vi "Node.vi"(8 "error in (no error)":errorcluster, 11 "Node Ptr":T1 format="%.0x") -> (0 "error out":errorcluster)   [LabVIEW 2016, in "PXImc Custom Device System Explorer.lvlib"]
uses:
  PXImc Custom Device System Explorer.lvlib
  <vilib>/NI Veristand/Custom Device API/Custom Device Item Ref.ctl
  Shared/Constants.vi
  <vilib>/NI Veristand/Custom Device API/Get Item Property (Variant).vi
  <vilib>/NI Veristand/Custom Device API/Set Item Property (Variant).vi
  <vilib>/NI VeriStand/Custom Device API/Custom Device API.lvlib
  Shared/PXImc Custom Device Shared.lvlib
panel:
  out "Imported Channels":string[][](table)
  out "Local Channels":string[][](table)
  out "PXImc Resource Name":string
  in  "Connection Timeout (s)":dbl
  in  "Readers Buffer Size":u64
  in  "Configution Files Path":path
  in  "Update Configuration":bool
  in  "Header":cluster{"Section Name":string}={"Section Name"="Custom Device Item Settings"}
  in  "Description":string
  in  "Name":string
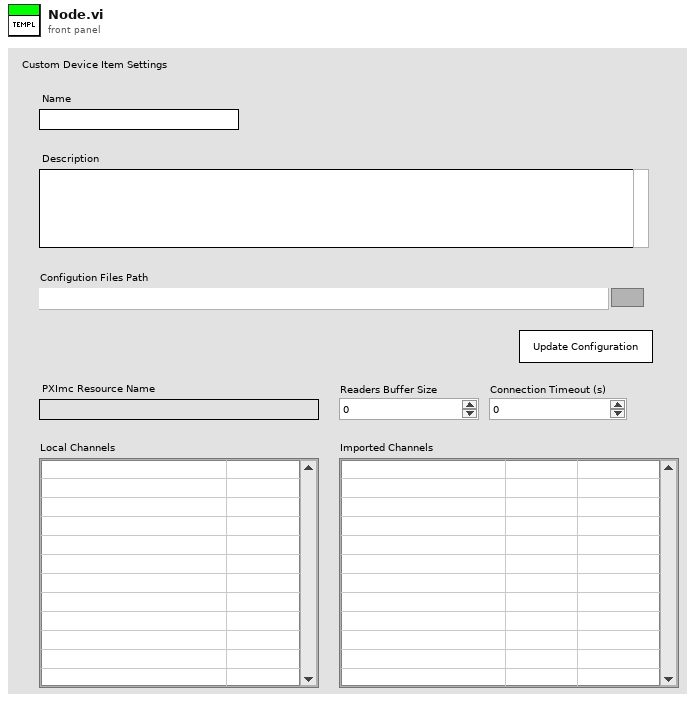
[diagram p1: front panel]
types:
  T1 = typedef "Custom Device API.lvlib/Custom Device Item Ref.ctl" = u64
  T2 = typedef "Custom Device API.lvlib/Custom Device Item Info.ctl" = cluster{"Name":string, "Is Channel":bool, "GUID":string, "Is Waveform":bool}
  T3 = typedef "PXImc Custom Device Shared.lvlib/Compiled.Settings.ctl" = cluster{"Target Type":T4, "Router Properties":T5, "Node Data":T10, "Configuration Folder Path":path}
  T4 = typedef "PXImc Router.lvlib/Target Type.ctl" = enum16{"Router", "Node"}
  T5 = typedef "PXImc Router.lvlib/Router - Configuration.ctl" = cluster{"Target Type":T4, "Master Table Ref":refnum<data-value>, "Master Table Size (Bytes)":u32, "Node Properties":T6[], "Router - PXImc Properties":T8}
  T6 = typedef "PXImc Router.lvlib/Node Block R-W Properties.ctl" = cluster{"Node ID":u32, "# Reading Blocks":u32, "Node Writing Block":T7, "Node Reading Blocks":T7[]}
  T7 = typedef "PXImc Router.lvlib/Block Properties.ctl" = cluster{"Offset":u32, "Size (Bytes)":u32}
  T8 = typedef "PXImc Router.lvlib/Router - PXImc Properties.ctl" = cluster{"PXImc Cards Properties":T9[], "Connection Timeout (s)":dbl, "Readers Buffer Size":u64}
  T9 = typedef "PXImc Router.lvlib/Router - PXImc Card Properties.ctl" = cluster{"PXImc Resource Name":string, "Reader - PXImc Session Ref":refnum<k21>, "Writer - PXImc Session Ref":refnum<k21>, "Reader Conn ID":u16, "Writer Conn ID":u16}
  T10 = typedef "PXImc Router.lvlib/Node Data.ctl" = cluster{"Node Name":string, "PXImc Parameters":T11, "Local Data":T12, "Imported Data":T15}
  T11 = typedef "PXImc Router.lvlib/Node - PXImc Parameters.ctl" = cluster{"Resource Name":string, "Connection Timeout (s)":dbl, "Readers Buffer Size":u64, "Node PXImc Reader Conn Id":u16, "Node PXImc Writer Conn Id":u16, "Writer PXImc Session":refnum<k21>, "Reader PXImc Session":refnum<k21>}
  T12 = typedef "PXImc Router.lvlib/Node - Writer Data.ctl" = cluster{"Noder ID":u32, "Byte Buffer Ref":refnum<class "Byte Buffer.lvclass">, "Master Table Offest":u32, "Byte Buffer Size":u32, "Node Local Channels":T13[], "Node Local Channels Table":string[][]}
  T13 = typedef "PXImc Router.lvlib/Node Ch Properties.ctl" = cluster{"Name":string, "Value":dbl, "Data Type":T14}
  T14 = typedef "PXImc Router.lvlib/Data Type.ctl" = enum16{"Boolean", "SGL", "DBL", "I8", "I16", "I32", "I64", "U8", "U16", "U32", "U64"}
  T15 = typedef "PXImc Router.lvlib/Node - Readers Data.ctl" = cluster{"Byte Buffer Ref":refnum<class "Byte Buffer.lvclass">, "Byte Buffer Size":u64, "Readers Data Array":T16[], "Node Imported Channels Table":string[][]}
  T16 = typedef "PXImc Router.lvlib/Node - Reader Data.ctl" = cluster{"Noder ID":u32, "Master Table Offest":u32, "Byte Buffer Size":u64, "Node Imported Channels":T13[]}
  T17 = typedef "Custom Device API.lvlib/Custom Device Commands.ctl" = enum16{"Default", "Item renamed", "Shutdown", "Dynamic button pressed"}
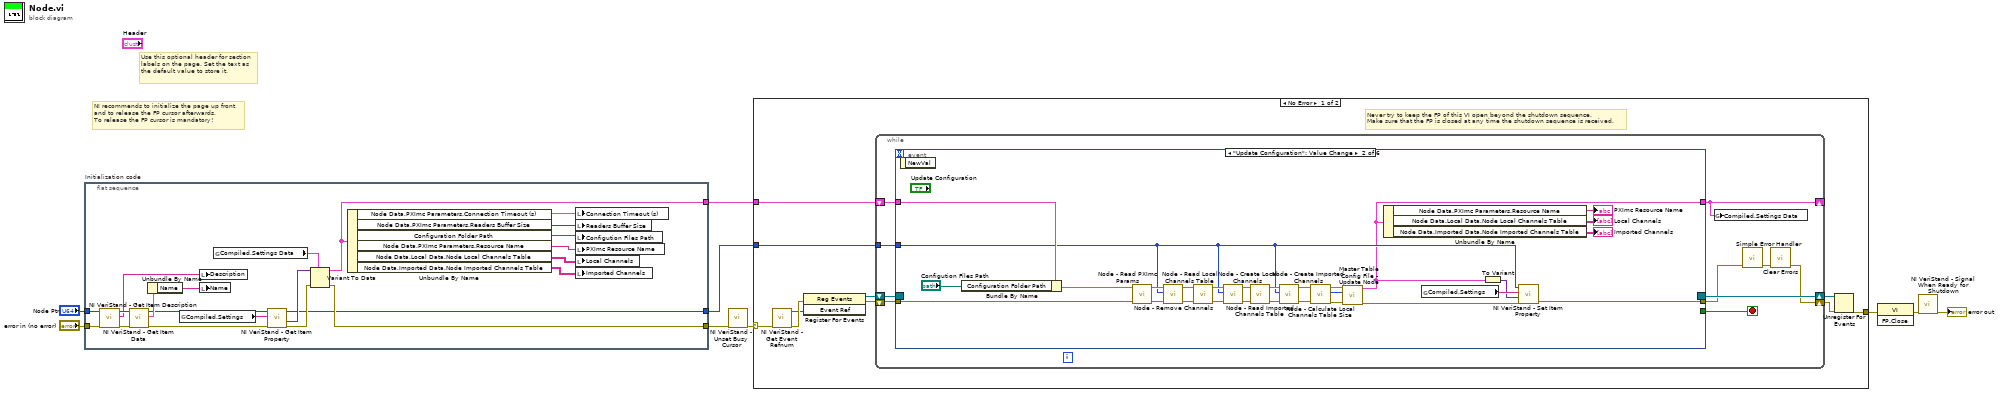
[diagram p0: block diagram]
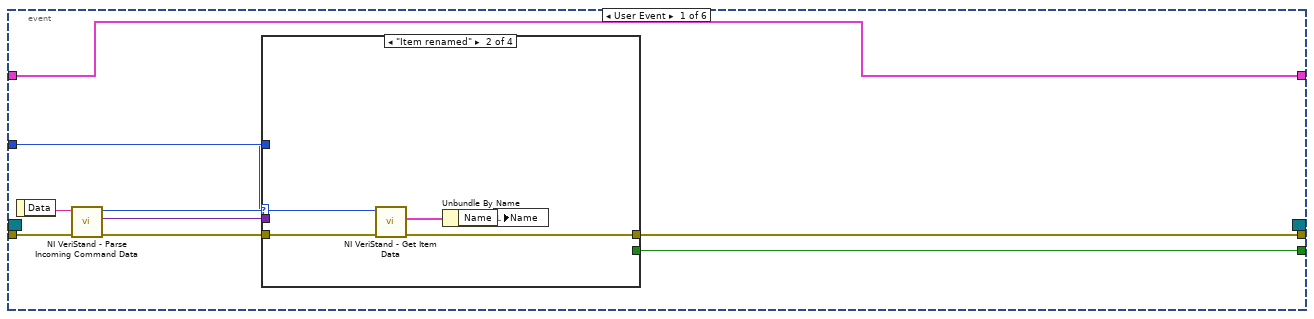
[diagram p2: hidden frame]
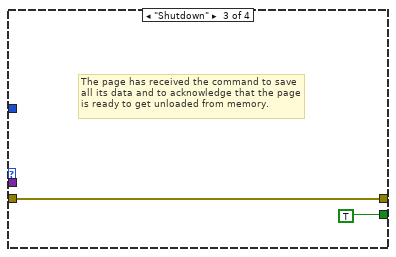
[diagram p4: hidden frame]
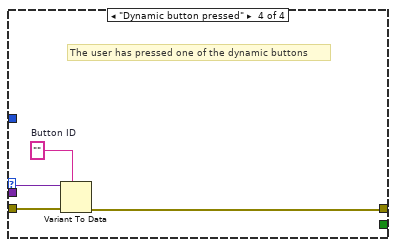
[diagram p5: hidden frame]
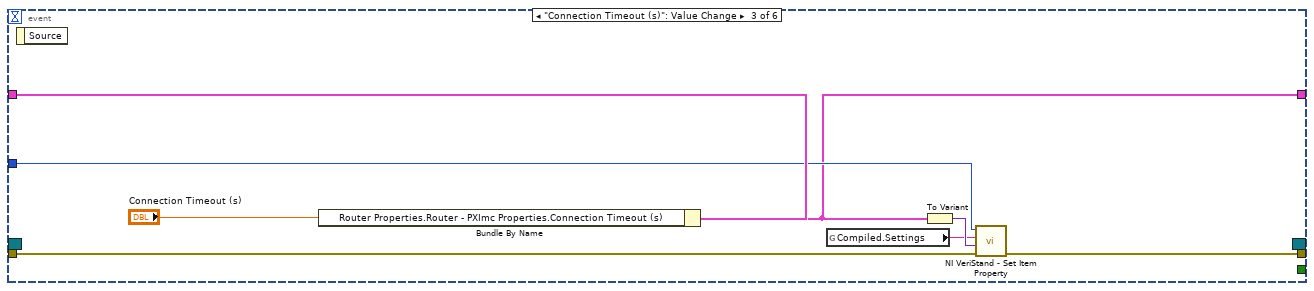
[diagram p6: hidden frame]
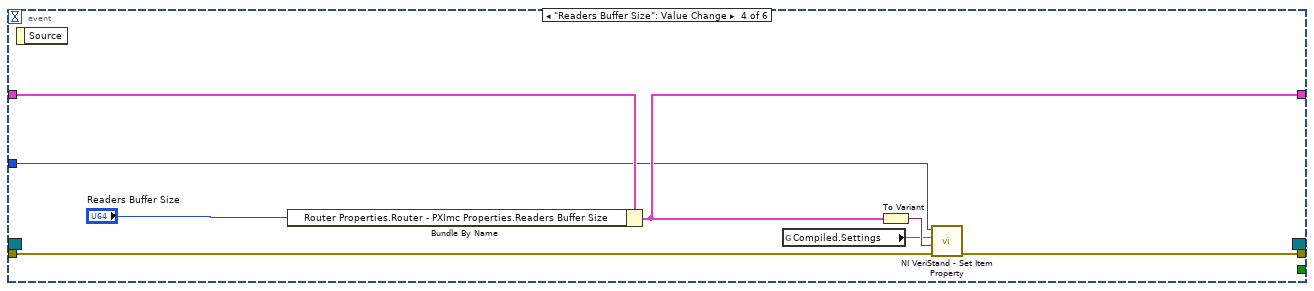
[diagram p7: hidden frame]
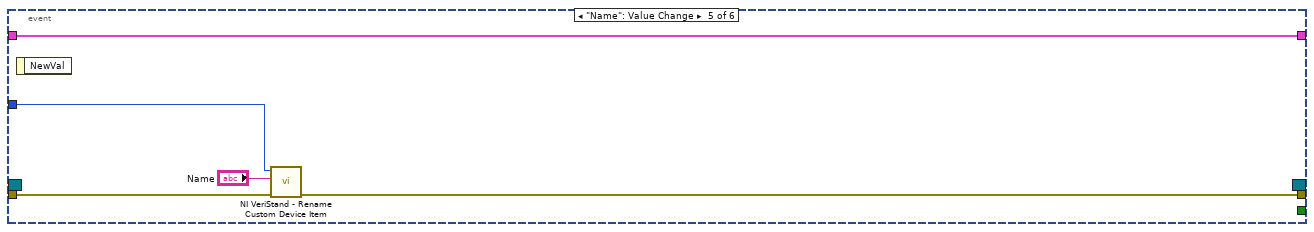
[diagram p8: hidden frame]
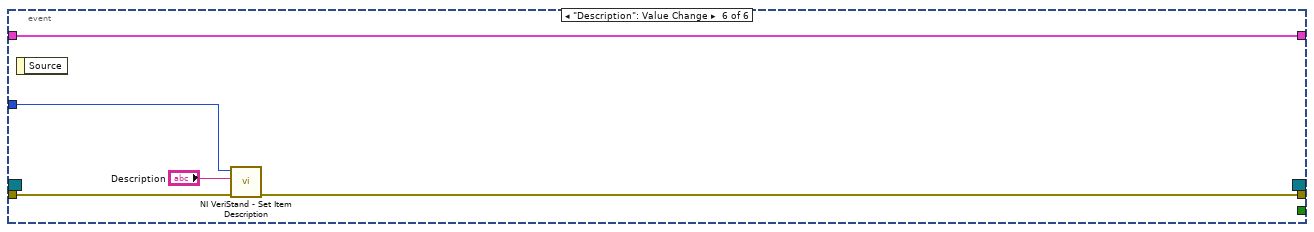
[diagram p9: hidden frame]
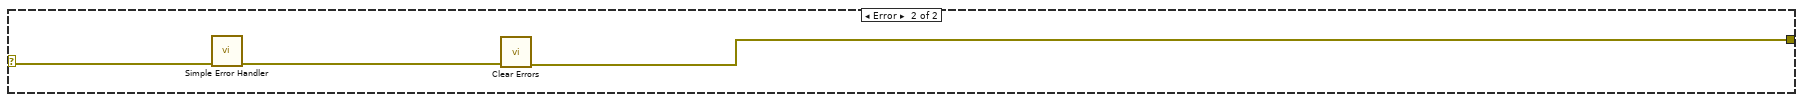
[diagram p10: hidden frame]
diagram:
  # "Use this optional header for section labels on the page. Set the text as the default value to store it."
  # "NI recommends to initialize the page up front\nand to release the FP cursor afterwards.\nTo release the FP cursor is mandatory!"
  n1 = flat-sequence "Initialization code" {
    tunnel: "error in (no error)" -> [w30]
    tunnel: "Node Ptr" -> [w29]
    tunnel: [w16] -> w5
    tunnel: [w15] -> w2
    tunnel: [w14] -> w1
    frame #0 {
      n2 = call <vilib>:"NI VeriStand - Get Item Description.vi"("error in (no error)"=w30, "Item Ref in"=w29) -> ("error out"=w27:errorcluster, "Description"=w28:string, "Item Ref out"=w31:T1)  [unwired: 7 out]
      n3 = call <vilib>:"NI VeriStand - Get Item Data.vi"("error in (no error)"=w27, "Item Ref in"=w31) -> ("error out"=w17:errorcluster, "Item Info"=w26:T2, "Item Ref out"=w18:T1)  [unwired: 7 out]
      n4 = Unbundle By Name(w26) -> ("Name"=w13:string)
      n5 = global read "Constants.vi" "Compiled.Settings"() -> (w19:string)
      n6 = local write "Description"(w28) -> ()
      n7 = local write "Name"(w13) -> ()
      n8 = global read "Constants.vi" "Compiled.Settings Data"() -> (w12:T3)
      n9 = call-poly <vilib>:"NI VeriStand - Get Item Property.vi"("error in (no error)"=w17, "Property Name"=w19, "Item Ref in"=w18) -> ("error out"=w20:errorcluster, "Value"=w21:variant, "Item Ref out"=w15:T1)  [unwired: 5 in, 1 out]
      n10 = Variant To Data(error in=w20, type=w12, Variant=w21) -> (data=w14:T3, error out=w16:errorcluster)
      n11 = Unbundle By Name(w14) -> ("Node Data.PXImc Parameters.Connection Timeout (s)"=w22:dbl, "Node Data.PXImc Parameters.Readers Buffer Size"=w23:u64, "Configuration Folder Path"=w24:path, "Node Data.PXImc Parameters.Resource Name"=w25:string, "Node Data.Local Data.Node Local Channels Table"=w11:string[][], "Node Data.Imported Data.Node Imported Channels Table"=w10:string[][])
      n12 = local write "Connection Timeout (s)"(w22) -> ()
      n13 = local write "Readers Buffer Size"(w23) -> ()
      n14 = local write "Configution Files Path"(w24) -> ()
      n15 = local write "PXImc Resource Name"(w25) -> ()
      n16 = local write "Local Channels"(w11) -> ()
      n17 = local write "Imported Channels"(w10) -> ()
    }
  }
  n18 = call <vilib>:"NI VeriStand - Unset Busy Cursor.vi"("error in (no error)"=w5) -> ("error out"=w4:errorcluster)  [unwired: 10 out]
  n19 = case shown="No Error" w4 {
    selector: w4 -> [w33 w129]
    tunnel: [w38 w127] -> w9
    tunnel: w2 -> [w34 _]
    tunnel: w1 -> [w32 _]
    frame No Error {
      # "Never try to keep the FP of this VI open beyond the shutdown sequence.\nMake sure that the FP is closed at any time the shutdown sequence is received."
      n20 = call <vilib>:"NI VeriStand - Get Event Refnum.vi"("error in (no error)"=w33) -> ("error out"=w41:errorcluster, "Event Ref"=w37:refnum<user-event>)  [unwired: 9 out]
      n21 = register-events(error in=w41, w37) -> (reference out=w35:refnum<event-registration>, error out=w36:errorcluster)  [unwired: 1 in]
      n22 = while {
        tunnel: w34 -> [w47]
        shift-right: [w44] -> w39
        shift-left: w36 -> [w50]
        shift-right: [w51] -> w40
        shift-left: w35 -> [w49]
        shift-right: [w42] -> _
        shift-left: w32 -> [w43]
        stop <- w48 stop-if-true
        n23 = event shown="[1] \"Update Configuration\": Value Change" {
          selector: w49 -> [_ _ _ _ _ _]
          dyn-events: [_ _ _ _ _ _] -> w51
          timeout: _ -> [_ _ _ _ _ _]
          tunnel: w50 -> [w60 w93 w103 w110 w121 w125]
          tunnel: [w56 _ _ _ _ _] -> w48
          tunnel: [w55 w98 w102 w109 w120 w124] -> w46
          tunnel: w47 -> [w54 w82 w104 w111 w119 w126]
          tunnel: w43 -> [w52 w97 w106 w114 w117 w122]
          tunnel: [w52 w74 w101 w112 w117 w122] -> w42
          event User Event {
            n24 = event-data() -> ("Data"=w59:string)  [unwired: 1 out]
            n25 = call <vilib>:"NI VeriStand - Parse Incoming Command Data.vi"("error in (no error)"=w60, "Incoming data"=w59) -> ("error out"=w58:errorcluster, "Outgoing data"=w53:variant, "Action"=w57:T17)  [unwired: 7 out]
            n26 = case shown="\"Item renamed\"" w57 {
              tunnel: w58 -> [w61 w66 w67 w72]
              tunnel: [_ _ TRUE _] -> w56
              tunnel: [w61 w63 w67 w69] -> w55
              tunnel: w54 -> [_ w65 _ _]
              tunnel: w53 -> [_ _ _ w71]
              frame "Default", Default {
              }
              frame "Item renamed" {
                n27 = call <vilib>:"NI VeriStand - Get Item Data.vi"("error in (no error)"=w66, "Item Ref in"=w65) -> ("error out"=w63:errorcluster, "Item Info"=w64:T2)  [unwired: 8 out]
                n28 = Unbundle By Name(w64) -> ("Name"=w62:string)
                n29 = local write "Name"(w62) -> ()
              }
              frame "Shutdown" {
                # "The page has received the command to save all its data and to acknowledge that the page is ready to get unloaded from memory."
              }
              frame "Dynamic button pressed" {
                w70 = ""  # Button ID
                # "The user has pressed one of the dynamic buttons"
                n30 = Variant To Data(error in=w72, type=w70, Variant=w71) -> (error out=w69:errorcluster)  [unwired: 1 out]
              }
            }
          }
          event "Update Configuration": Value Change {
            n31 = event-data() -> ()  [unwired: 2 out]
            n32 = Bundle By Name(cluster=w97, "Configuration Folder Path"="Configution Files Path") -> (w94:T3)
            n33 = call "Node - Read PXImc Params.vi"("error in (no error)"=w93, "Compiled.Settings In"=w94) -> ("error out"=w81:errorcluster, "Compiled.Settings Out"=w84:T3)  [unwired: 8 in]
            n34 = call "Node - Remove Channels.vi"("error in (no error)"=w81, "Node Ptr In"=w82, "Compiled.Settings In"=w84) -> ("error out"=w80:errorcluster, "Compiled.Settings Out"=w83:T3)  [unwired: 6 in, 1 out]
            n35 = call "Node - Read Local Channels Table.vi"("error in (no error)"=w80, "Compiled.Settings In"=w83) -> ("error out"=w91:errorcluster, "Compiled.Settings Out"=w92:T3)  [unwired: 8 in]
            n36 = call "Node - Create Local Channels.vi"("error in (no error)"=w91, "Node Ptr In"=w82, "Compiled.Settings In"=w92) -> ("error out"=w89:errorcluster, "Compiled.Settings Out"=w90:T3)  [unwired: 6 in, 1 out]
            n37 = call "Node - Read Imported Channels Table.vi"("error in (no error)"=w89, "Compiled.Settings In"=w90) -> ("error out"=w87:errorcluster, "Compiled.Settings Out"=w88:T3)  [unwired: 8 in]
            n38 = call "Node - Create Imported Channels.vi"("error in (no error)"=w87, "Node Ptr In"=w82, "Compiled.Settings In"=w88) -> ("error out"=w75:errorcluster, "Compiled.Settings Out"=w76:T3)  [unwired: 6 in, 1 out]
            n39 = call "Node - Calculate Local Channels Table Size.vi"("error in (no error)"=w75, "Compiled.Settings In"=w76) -> ("error out"=w79:errorcluster, "Local Channels Table Size Out"=w78:u64, "Compiled.Settings Out"=w77:T3)  [unwired: 7 in]
            n40 = call "Master Table Config File - Update Node.vi"("error in (no error)"=w79, "Local Channels Table Size In"=w78, "Compiled.Settings In"=w77) -> ("error out"=w73:errorcluster, "Compiled.Settings Out"=w74:T3)  [unwired: 7 in]
            n41 = Unbundle By Name(w74) -> ("Node Data.PXImc Parameters.Resource Name"=→"PXImc Resource Name":string, "Node Data.Local Data.Node Local Channels Table"=→"Local Channels":string[][], "Node Data.Imported Data.Node Imported Channels Table"=→"Imported Channels":string[][])
            n42 = global read "Constants.vi" "Compiled.Settings"() -> (w100:string)
            n43 = To Variant(anything=w74) -> (Variant=w99:variant)
            n44 = call-poly <vilib>:"NI VeriStand - Set Item Property.vi"("error in (no error)"=w73, "Value"=w99, "Property Name"=w100, "Item Ref in"=w82) -> ("error out"=w98:errorcluster)  [unwired: 5 in, 2 out]
          }
          event "Connection Timeout (s)": Value Change {
            n45 = event-data() -> ()  [unwired: 2 out]
            n46 = Bundle By Name(cluster=w106, "Router Properties.Router - PXImc Properties.Connection Timeout (s)"="Connection Timeout (s)") -> (w101:T3)
            n47 = global read "Constants.vi" "Compiled.Settings"() -> (w107:string)
            n48 = To Variant(anything=w101) -> (Variant=w108:variant)
            n49 = call-poly <vilib>:"NI VeriStand - Set Item Property.vi"("error in (no error)"=w103, "Value"=w108, "Property Name"=w107, "Item Ref in"=w104) -> ("error out"=w102:errorcluster)  [unwired: 5 in, 2 out]
          }
          event "Readers Buffer Size": Value Change {
            n50 = event-data() -> ()  [unwired: 2 out]
            n51 = Bundle By Name(cluster=w114, "Router Properties.Router - PXImc Properties.Readers Buffer Size"="Readers Buffer Size") -> (w112:T3)
            n52 = global read "Constants.vi" "Compiled.Settings"() -> (w115:string)
            n53 = To Variant(anything=w112) -> (Variant=w116:variant)
            n54 = call-poly <vilib>:"NI VeriStand - Set Item Property.vi"("error in (no error)"=w110, "Value"=w116, "Property Name"=w115, "Item Ref in"=w111) -> ("error out"=w109:errorcluster)  [unwired: 5 in, 2 out]
          }
          event "Name": Value Change {
            n55 = event-data() -> ()  [unwired: 2 out]
            n56 = call <vilib>:"NI VeriStand - Rename Custom Device Item.vi"("error in (no error)"=w121, "New Name"="Name", "Item Ref in"=w119) -> ("error out"=w120:errorcluster)  [unwired: 1 in, 7 out]
          }
          event "Description": Value Change {
            n57 = event-data() -> ()  [unwired: 2 out]
            n58 = call <vilib>:"NI VeriStand - Set Item Description.vi"("error in (no error)"=w125, "Description"="Description", "Item Ref in"=w126) -> ("error out"=w124:errorcluster)  [unwired: 8 out]
          }
        }
        n59 = global write "Constants.vi" "Compiled.Settings Data"(w42) -> ()
        n60 = call <vilib>:"Simple Error Handler.vi"("error in (no error)"=w46) -> ("error out"=w45:errorcluster)  [unwired: 1 in, 7 out]
        n61 = call <vilib>:"Clear Errors.vi"("error in (no error)"=w45) -> ("error out"=w44:errorcluster)  [unwired: 1 in, 5 out]
      }
      n62 = Unregister For Events(event registration refnum=w40, error in=w39) -> (error out=w38:errorcluster)
    }
    frame Error {
      n63 = call <vilib>:"Simple Error Handler.vi"("error in (no error)"=w129) -> ("error out"=w128:errorcluster)  [unwired: 1 in, 7 out]
      n64 = call <vilib>:"Clear Errors.vi"("error in (no error)"=w128) -> ("error out"=w127:errorcluster)  [unwired: 1 in, 5 out]
    }
  }
  n65 = invoke class="VI" method="FP.Close"(error in=w9) -> (error out=w8:errorcluster)  [unwired: 2 in, 2 out]
  n66 = call <vilib>:"NI VeriStand - Signal When Ready for Shutdown.vi"("error in (no error)"=w8) -> ("error out"=→"error out":errorcluster)  [unwired: 10 out]
